vi "Step Core.vi"(8 "error in (no error)":errorcluster, 11 "Abort Keep Alive in":refnum<class "Abort Keep Alive.lvclass">) -> (0 "error out":errorcluster, 3 "Abort Keep Alive out":refnum<class "Abort Keep Alive.lvclass">)   [LabVIEW 2018, in "Abort Keep Alive.lvlib" / "Abort Keep Alive.lvclass"]
uses:
  Abort Keep Alive.lvclass
  Plugins/Measurement Interface.lvlibp/Measurement Interface.lvclass
  C:/Sequence Automation/Plugins/Measurement Interface.lvlibp/Measurement Interface.lvclass
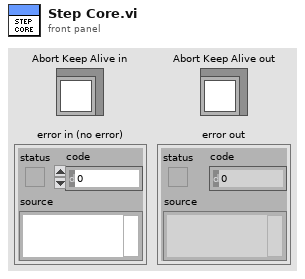
[diagram p1: front panel]
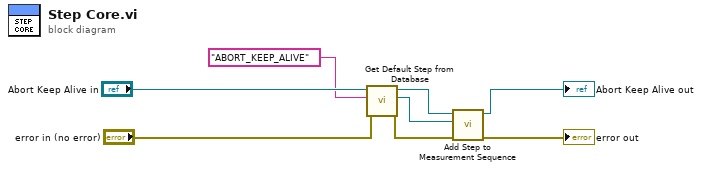
[diagram p0: block diagram]
diagram:
  n1 = call "Get Default Step from Database.vi"("error in (no error)"="error in (no error)", "Default Step"="ABORT_KEEP_ALIVE", "Measurement Interface in"="Abort Keep Alive in") -> ("error out"=w5:errorcluster, "Cloned Step"=w1:refnum<k7>, "Measurement Interface out"=w3:refnum<class "Abort Keep Alive.lvclass">)  [unwired: 6 in]
  n2 = call "Add Step to Measurement Sequence.vi"("error in (no error)"=w5, "Step to Add"=w1, "Measurement Interface in"=w3) -> ("error out"=→"error out":errorcluster, "Measurement Interface out"=→"Abort Keep Alive out":refnum<class "Abort Keep Alive.lvclass">)  [unwired: 7 in]
